vi "WebCommands.vi"(0 "Analyte":refnum<vi>, 1 "Bias":refnum<vi>, 2 "MessageQueues":T1, 5 "channels":refnum<vi>, 7 "buffer":refnum<vi>, 9 "notes":refnum<vi>, 11 "waferChip":refnum<vi>, 12 "experiment":refnum<vi>, 13 "reference 8":refnum<vi>) -> (6 "frequency":dbl=20.0, 8 "error out 2":errorcluster, 15 "error out":errorcluster)   [LabVIEW 2024]
uses:
  MessageQueues.ctl
  <vilib>/httpClient/ClientHandle.ctl
  experimentDefinition.ctl
  <vilib>/httpClient/LabVIEWHTTPClient.lvlib
  <vilib>/wsapi/NI_WebServices.lvlib
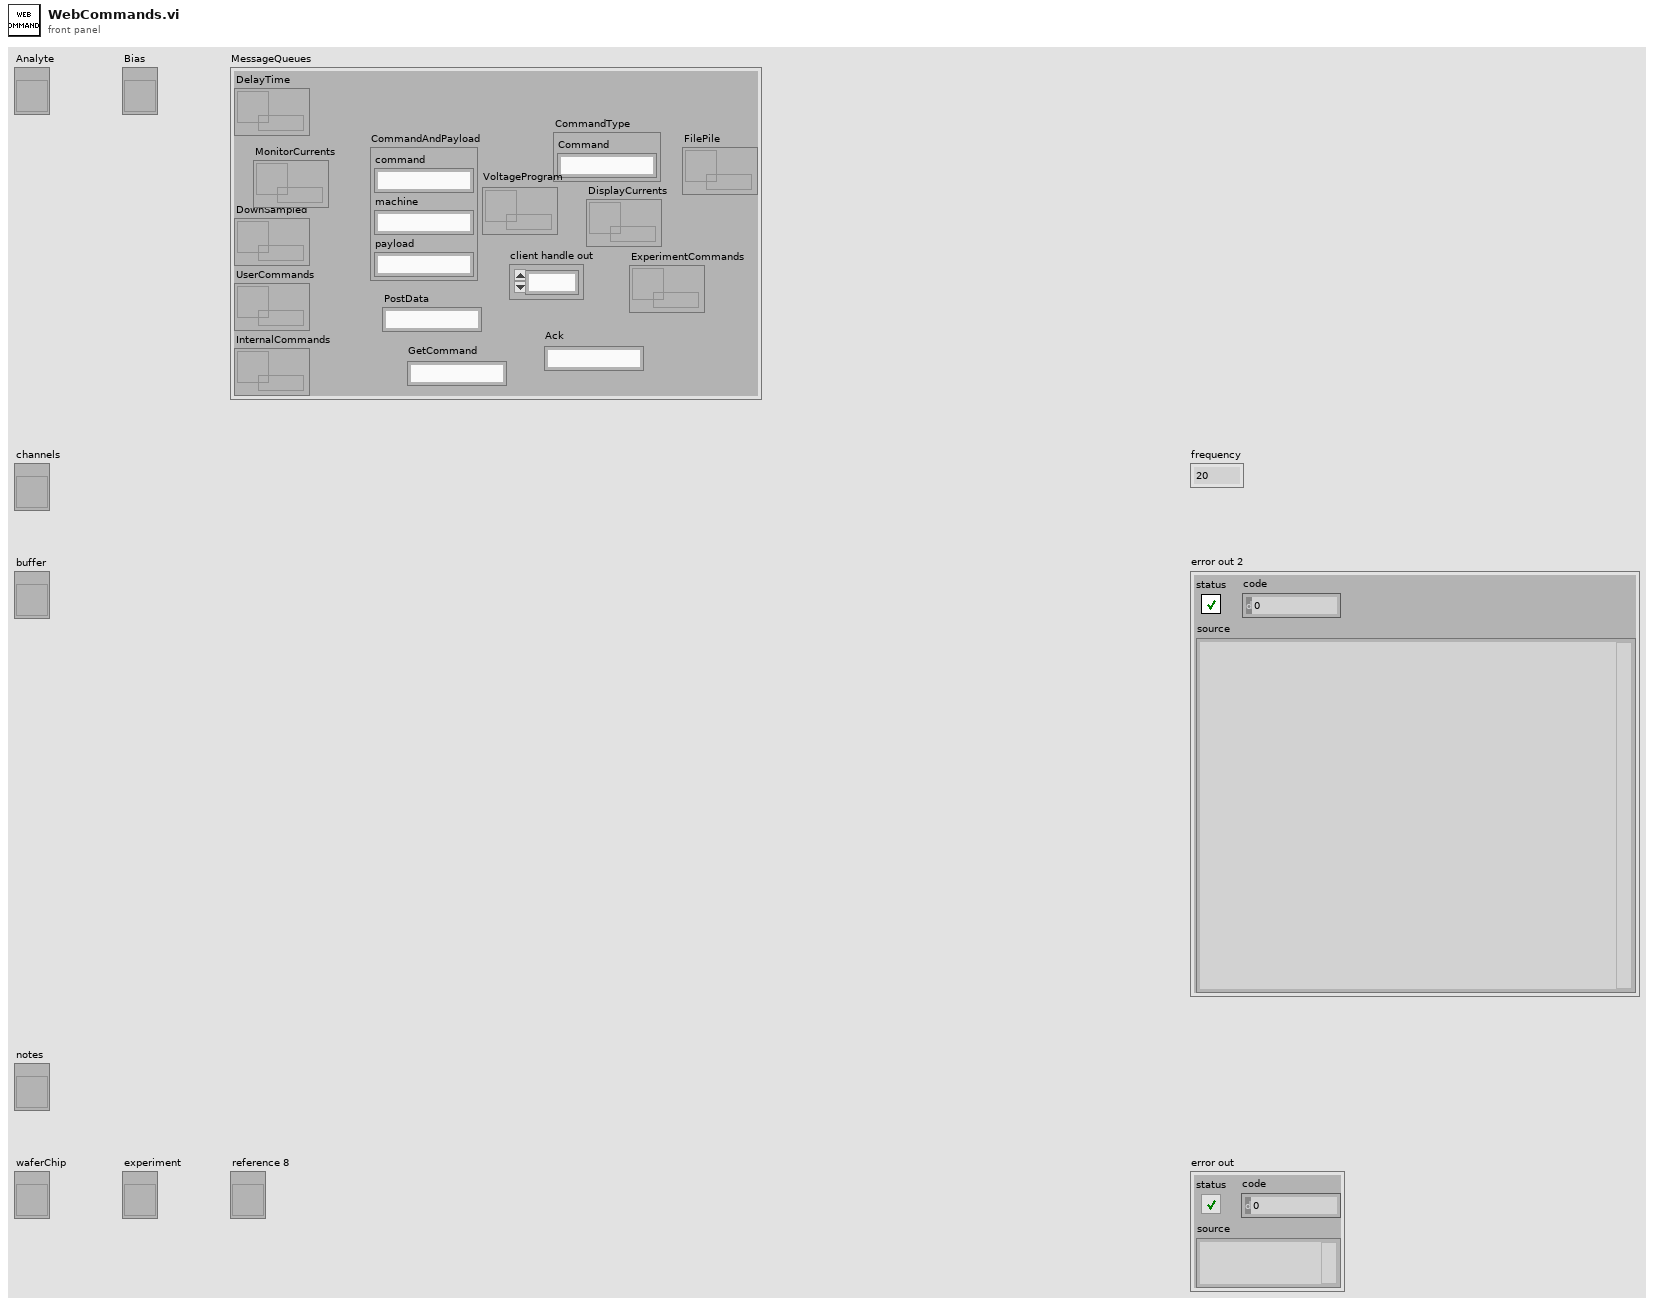
[diagram p1: front panel]
types:
  T1 = typedef "MessageQueues.ctl" = cluster{"DelayTime":refnum<queue>, "DownSampled":refnum<queue>, "UserCommands":refnum<queue>, "InternalCommands":refnum<queue>, "CommandType":cluster{"Command":string}, "CommandAndPayload":cluster{"command":string, "machine":string, "payload":string}, "client handle out":T2, "PostData":string, "GetCommand":string, "Ack":string, "VoltageProgram":refnum<queue>, "ExperimentCommands":refnum<queue>, "DisplayCurrents":refnum<queue>, "MonitorCurrents":refnum<queue>, "FilePile":refnum<queue>}
  T2 = typedef "LabVIEWHTTPClient.lvlib/ClientHandle.ctl" = refnum<k1>
  T3 = cluster{"command":string, "machine":string, "payload":string}
  T4 = typedef "experimentDefinition.ctl" = cluster{"id":i32, "primary":string, "secondary":string, "steps":cluster{"id":i32, "macro":cluster{"id":i32, "primary":string, "secondary":string, "rows":cluster{"id":i32, "analyte1":string, "analyte2":string, "volume1":string, "volume2":string, "speed1":string, "speed2":string, "time":string, "bias":string, "measurement":string}[]}}[]}
  T5 = cluster{"channels":string, "analyte":string, "notes":string, "buffer":string, "experiment":string, "waferChip":string}
  T6 = cluster{"duration":dbl, "bias":dbl, "frequency":dbl}
  T7 = cluster{"id":i32, "macro":cluster{"id":i32, "primary":string, "secondary":string, "rows":cluster{"id":i32, "analyte1":string, "analyte2":string, "volume1":string, "volume2":string, "speed1":string, "speed2":string, "time":string, "bias":string, "measurement":string}[]}}[]
  T8 = cluster{"id":i32, "analyte1":string, "analyte2":string, "volume1":string, "volume2":string, "speed1":string, "speed2":string, "time":string, "bias":string, "measurement":string}[]
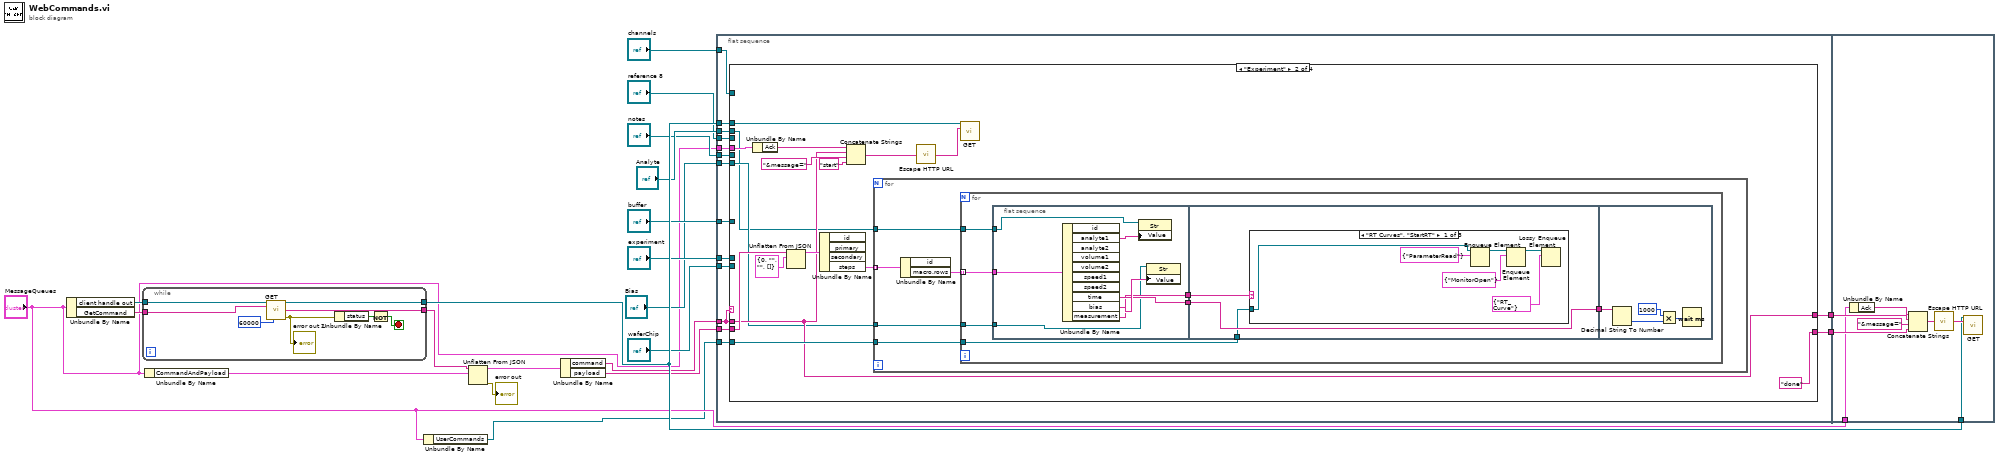
[diagram p0: block diagram]
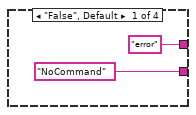
[diagram p2: hidden frame]
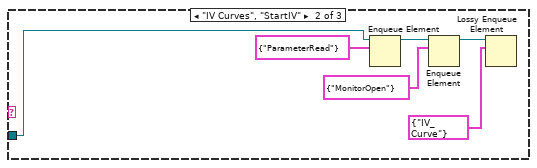
[diagram p3: hidden frame]
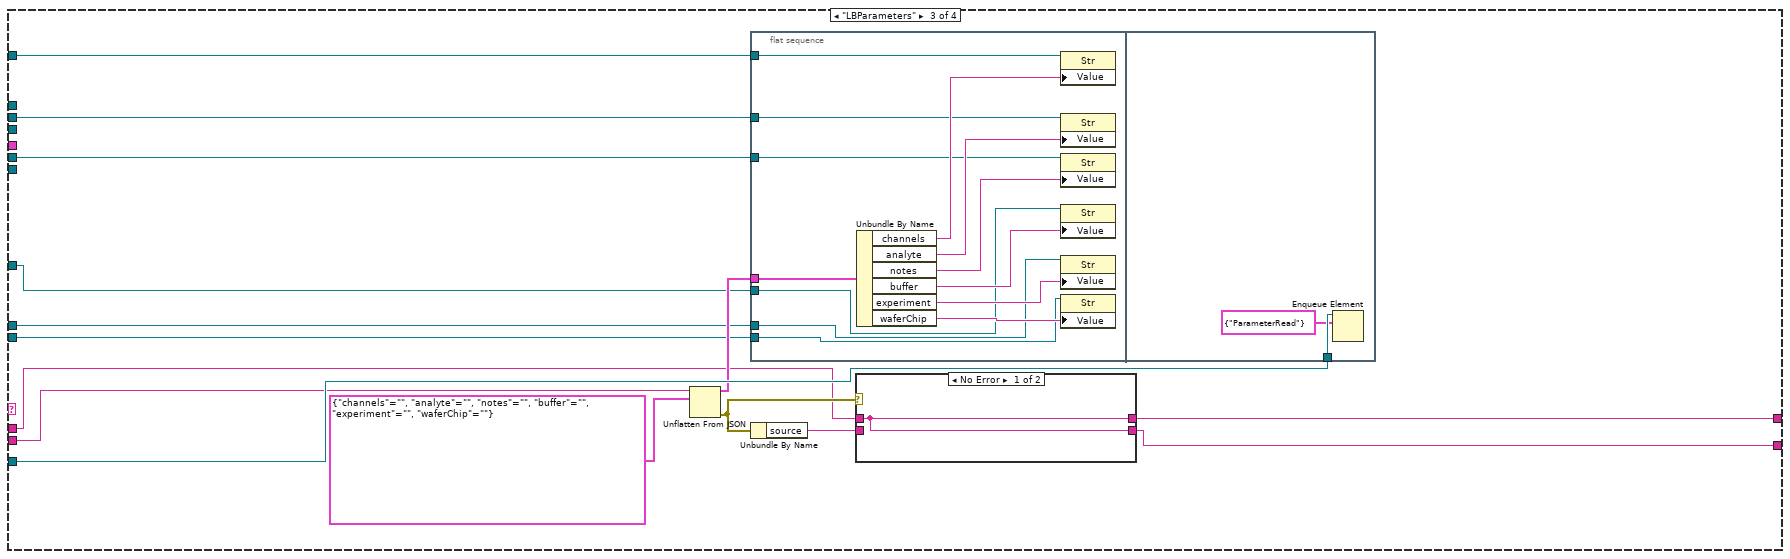
[diagram p5: hidden frame]
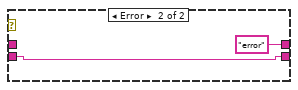
[diagram p6: hidden frame]
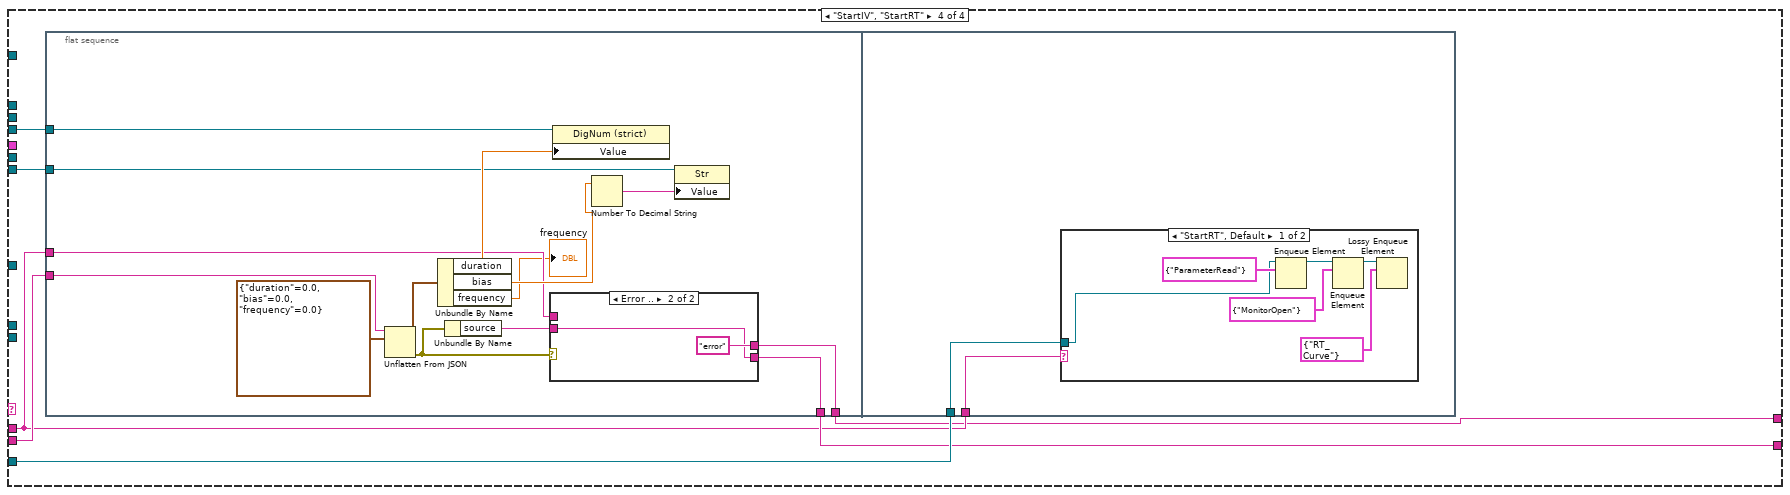
[diagram p7: hidden frame]
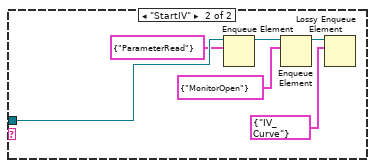
[diagram p9: hidden frame]
diagram:
  n1 = Unbundle By Name("MessageQueues") -> ("client handle out"=w18:T2, "GetCommand"=w19:string)
  n2 = while {
    tunnel: [w28] -> w11
    tunnel: w19 -> [w24]
    tunnel: w18 -> [w23]
    tunnel: [w22] -> w16
    stop <- w25 stop-if-true
    n3 = call <vilib>:"GET.vi"("client handle"=w23, "url"=w24, "timeout (10000)"=60000) -> ("client handle out"=w22:T2, "body"=w28:string, "error out"=w27:errorcluster)  [unwired: 9 in, 1 out]
    "error out 2" <- w27
    n4 = Unbundle By Name(w27) -> ("status"=w26:bool)
    n5 = Not(x=w26) -> (.not. x?=w25:bool)
  }
  n6 = Unbundle By Name("MessageQueues") -> ("CommandAndPayload"=w17:T3)
  n7 = Unbundle By Name("MessageQueues") -> ("UserCommands"=w1:refnum<queue>)
  n8 = Unflatten From JSON(JSON string=w11, type and defaults=w17) -> (value=w12:T3, error out=→"error out":errorcluster)  [unwired: 5 in]
  n9 = Unbundle By Name(w12) -> ("command"=w14:string, "payload"=w13:string)
  n10 = flat-sequence {
    tunnel: w13 -> [w44]
    tunnel: w1 -> [w43]
    tunnel: w14 -> [w42]
    tunnel: [w41] -> w21
    tunnel: [w40] -> w20
    tunnel: "MessageQueues" -> [w39]
    tunnel: w16 -> [w38]
    tunnel: "channels" -> [w37]
    tunnel: "Analyte" -> [w36]
    tunnel: "buffer" -> [w35]
    tunnel: "notes" -> [w34]
    tunnel: "waferChip" -> [w33]
    tunnel: "experiment" -> [w32]
    tunnel: "reference 8" -> [w31]
    tunnel: "Bias" -> [w30]
    tunnel: w21 -> [w179]
    tunnel: w20 -> [w175]
    tunnel: "MessageQueues" -> [w174]
    tunnel: w16 -> [w173]
    frame #0 {
      n11 = case shown="\"Experiment\"" w42 {
        tunnel: w43 -> [_ w58 w115 w139]
        tunnel: w44 -> [_ w61 w113 w140]
        tunnel: w42 -> [_ w54 w110 w137]
        tunnel: ["NoCommand" ("source") "done" ("source") w107 w138] -> w41
        tunnel: ["error" ("command") w54 w109 w136] -> w40
        tunnel: w39 -> [_ w53 _ _]
        tunnel: w38 -> [_ w50 _ _]
        tunnel: w37 -> [_ _ w106 _]
        tunnel: w36 -> [_ w47 w105 _]
        tunnel: w35 -> [_ _ w104 _]
        tunnel: w34 -> [_ _ w103 _]
        tunnel: w33 -> [_ _ w102 _]
        tunnel: w32 -> [_ _ w101 _]
        tunnel: w31 -> [_ _ _ w135]
        tunnel: w30 -> [_ w48 _ w134]
        frame "False", Default {
        }
        frame "Experiment" {
          n12 = Unbundle By Name(w53) -> ("Ack"=w49:string)
          n13 = Unflatten From JSON(JSON string=w61, type and defaults=T4 {"id"=0, "primary"="", "secondary"="", "steps"=[]}) -> (value=w60:T4)  [unwired: 5 in, 1 out]
          n14 = Unbundle By Name(w60) -> ("steps"=w59:T7)  [unwired: 3 out]
          n15 = Concatenate Strings(w49, w54, "&message=" ("string"), "start" ("string")) -> (w55:string)
          n16 = for {
            tunnel: w59 -> [w67] mode=indexing
            tunnel: w58 -> [w65]
            tunnel: w47 -> [w64]
            tunnel: w48 -> [w63]
            n17 = Unbundle By Name(w67) -> ("macro.rows"=w66:T8)  [unwired: 1 out]
            n18 = for {
              tunnel: w66 -> [w74] mode=indexing
              tunnel: w65 -> [w71]
              tunnel: w64 -> [w69]
              tunnel: w63 -> [w68]
              n19 = flat-sequence {
                tunnel: w74 -> [w81]
                tunnel: [w78] -> w73
                tunnel: [w77] -> w70
                tunnel: w69 -> [w76]
                tunnel: w68 -> [w75]
                tunnel: w73 -> [w84]
                tunnel: [w84] -> w72
                tunnel: w71 -> [w83]
                tunnel: w70 -> [w82]
                tunnel: w72 -> [w100]
                frame #0 {
                  n20 = Unbundle By Name(w81) -> ("analyte1"=w80:string, "time"=w78:string, "bias"=w79:string, "measurement"=w77:string)  [unwired: 6 out]
                  n21 = property class="Str"(reference=w76, "Value"=w80) -> ()  [unwired: 1 in, 2 out]
                  n22 = property class="Str"(reference=w75, "Value"=w79) -> ()  [unwired: 1 in, 2 out]
                }
                frame #1 {
                  n23 = case shown="\"RT Curves\", \"StartRT\"" w82 {
                    tunnel: w83 -> [w85 w96 _]
                    frame "RT Curves", "StartRT" {
                      n24 = Enqueue Element(queue=w85, element=cluster{"Command":string} {"Command"="ParameterRead"}) -> (queue out=w86:refnum<queue>)  [unwired: 2 in, 2 out]
                      n25 = Enqueue Element(queue=w86, element=cluster{"Command":string} {"Command"="MonitorOpen"}) -> (queue out=w88:refnum<queue>)  [unwired: 2 in, 2 out]
                      n26 = Lossy Enqueue Element(queue=w88, element=cluster{"Command":string} {"Command"="RT_Curve"}) -> ()  [unwired: 1 in, 4 out]
                    }
                    frame "IV Curves", "StartIV" {
                      n27 = Enqueue Element(queue=w96, element=cluster{"Command":string} {"Command"="ParameterRead"}) -> (queue out=w91:refnum<queue>)  [unwired: 2 in, 2 out]
                      n28 = Enqueue Element(queue=w91, element=cluster{"Command":string} {"Command"="MonitorOpen"}) -> (queue out=w93:refnum<queue>)  [unwired: 2 in, 2 out]
                      n29 = Lossy Enqueue Element(queue=w93, element=cluster{"Command":string} {"Command"="IV_Curve"}) -> ()  [unwired: 1 in, 4 out]
                    }
                    frame Default {
                    }
                  }
                }
                frame #2 {
                  n30 = Decimal String To Number(string=w100) -> (number=w99:i32)  [unwired: 2 in, 1 out]
                  n31 = Multiply(x=1000, y=w99) -> (x*y=w98:i32)
                  n32 = Wait (ms)(milliseconds to wait=w98) -> ()  [unwired: 1 out]
                }
              }
            }
          }
          n33 = call <vilib>:"Escape HTTP URL.vi"("unescaped string in"=w55) -> ("escaped string out"=w51:string)
          n34 = call <vilib>:"GET.vi"("client handle"=w50, "url"=w51) -> ()  [unwired: 10 in, 4 out]
        }
        frame "LBParameters" {
          n35 = Unflatten From JSON(JSON string=w113, type and defaults=T5 {"channels"="", "analyte"="", "notes"="", "buffer"="", "experiment"="", "waferChip"=""}) -> (value=w112:T5, error out=w111:errorcluster)  [unwired: 5 in]
          n36 = flat-sequence {
            tunnel: w112 -> [w128]
            tunnel: w106 -> [w121]
            tunnel: w105 -> [w120]
            tunnel: w104 -> [w119]
            tunnel: w103 -> [w118]
            tunnel: w102 -> [w117]
            tunnel: w101 -> [w116]
            tunnel: w115 -> [w130]
            frame #0 {
              n37 = Unbundle By Name(w128) -> ("channels"=w127:string, "analyte"=w126:string, "notes"=w125:string, "buffer"=w124:string, "experiment"=w123:string, "waferChip"=w122:string)
              n38 = property class="Str"(reference=w121, "Value"=w127) -> ()  [unwired: 1 in, 2 out]
              n39 = property class="Str"(reference=w120, "Value"=w126) -> ()  [unwired: 1 in, 2 out]
              n40 = property class="Str"(reference=w118, "Value"=w125) -> ()  [unwired: 1 in, 2 out]
              n41 = property class="Str"(reference=w119, "Value"=w124) -> ()  [unwired: 1 in, 2 out]
              n42 = property class="Str"(reference=w116, "Value"=w123) -> ()  [unwired: 1 in, 2 out]
              n43 = property class="Str"(reference=w117, "Value"=w122) -> ()  [unwired: 1 in, 2 out]
            }
            frame #1 {
              n44 = Enqueue Element(queue=w130, element=cluster{"Command":string} {"Command"="ParameterRead"}) -> ()  [unwired: 2 in, 3 out]
            }
          }
          n45 = Unbundle By Name(w111) -> ("source"=w108:string)
          n46 = case shown="No Error" w111 {
            tunnel: w110 -> [w131 _]
            tunnel: [w131 "error" ("command")] -> w109
            tunnel: w108 -> [_ w132]
            tunnel: [w131 w132] -> w107
            frame No Error {
            }
            frame Error {
            }
          }
        }
        frame "StartIV", "StartRT" {
          n47 = flat-sequence {
            tunnel: w140 -> [w153]
            tunnel: [w144] -> w138
            tunnel: w137 -> [w147]
            tunnel: [w146] -> w136
            tunnel: w135 -> [w142]
            tunnel: w134 -> [w141]
            tunnel: w137 -> [w159]
            tunnel: w139 -> [w158]
            frame #0 {
              n48 = Unflatten From JSON(JSON string=w153, type and defaults=T6 {"duration"=0.0, "bias"=0.0, "frequency"=0.0}) -> (value=w152:T6, error out=w148:errorcluster)  [unwired: 5 in]
              n49 = Unbundle By Name(w152) -> ("duration"=w150:dbl, "bias"=w151:dbl, "frequency"=→"frequency":dbl)
              n50 = Unbundle By Name(w148) -> ("source"=w145:string)
              n51 = case shown="Error .." w148 {
                tunnel: w147 -> [w155 _]
                tunnel: [w155 "error" ("command")] -> w146
                tunnel: w145 -> [_ w156]
                tunnel: [w155 w156] -> w144
                frame No Error {
                }
                frame Error {
                }
              }
              n52 = property class="DigNum (strict)"(reference=w142, "Value"=w150) -> ()  [unwired: 1 in, 2 out]
              n53 = Number To Decimal String(number=w151) -> (decimal integer string=w149:string)  [unwired: 1 in]
              n54 = property class="Str"(reference=w141, "Value"=w149) -> ()  [unwired: 1 in, 2 out]
            }
            frame #1 {
              n55 = case shown="\"StartRT\", Default" w159 {
                tunnel: w158 -> [w160 w171]
                frame "StartRT", Default {
                  n56 = Enqueue Element(queue=w160, element=cluster{"Command":string} {"Command"="ParameterRead"}) -> (queue out=w161:refnum<queue>)  [unwired: 2 in, 2 out]
                  n57 = Enqueue Element(queue=w161, element=cluster{"Command":string} {"Command"="MonitorOpen"}) -> (queue out=w163:refnum<queue>)  [unwired: 2 in, 2 out]
                  n58 = Lossy Enqueue Element(queue=w163, element=cluster{"Command":string} {"Command"="RT_Curve"}) -> ()  [unwired: 1 in, 4 out]
                }
                frame "StartIV" {
                  n59 = Enqueue Element(queue=w171, element=cluster{"Command":string} {"Command"="ParameterRead"}) -> (queue out=w166:refnum<queue>)  [unwired: 2 in, 2 out]
                  n60 = Enqueue Element(queue=w166, element=cluster{"Command":string} {"Command"="MonitorOpen"}) -> (queue out=w168:refnum<queue>)  [unwired: 2 in, 2 out]
                  n61 = Lossy Enqueue Element(queue=w168, element=cluster{"Command":string} {"Command"="IV_Curve"}) -> ()  [unwired: 1 in, 4 out]
                }
              }
            }
          }
        }
      }
    }
    frame #1 {
      n62 = Unbundle By Name(w174) -> ("Ack"=w172:string)
      n63 = Concatenate Strings(w172, w175, "&message=" ("string"), w179) -> (w177:string)
      n64 = call <vilib>:"Escape HTTP URL.vi"("unescaped string in"=w177) -> ("escaped string out"=w176:string)
      n65 = call <vilib>:"GET.vi"("client handle"=w173, "url"=w176) -> ()  [unwired: 10 in, 4 out]
    }
  }
